vi "Delete Image.vi"(8 "Error In":errorcluster, 11 "Image Object":T1={"Device ID"=0, "Memeroy ID"=0, "Image Parameters"={"Channel Order"=enum."CL_LUMINANCE (Grayscale)", "Dimension"={"Depth"=1, "Height"=1, "Width"=1}, "Data Type"=enum."32f", "Offset"={"X"=0, "Y"=0, "Z"=0}}} {"Image Parameters"."Dimension"."Width" min=1; "Image Parameters"."Dimension"."Height" min=1; "Image Parameters"."Dimension"."Depth" min=1}) -> (0 "Error Out":errorcluster, 3 "Device Out":T2)   [LabVIEW 2012]
doc: "Deletes allocated memory on a device. It is best to call this at the end to avoid memory fragmentation due to constantly allocating and deleting memory."
uses:
  Non-User VIs/Controls/Device ID.ctl
  Non-User VIs/Controls/Image Object.ctl
  Non-User VIs/Controls/Memory ID.ctl
  Non-User VIs/Controls/Image Parameters.ctl
  Non-User VIs/Images/Channel Order.ctl
  User Controls/Array Dimensions.ctl
  Non-User VIs/Images/Data Type.ctl
  User Controls/Offset.ctl
  Non-User VIs/Error Checking/Add Error Functional Global.vi
  OpenCLV x64.lvlib
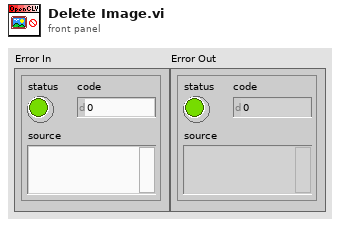
[diagram p1: front panel]
types:
  T1 = typedef "OpenCLV x64.lvlib/Image Object.ctl" = cluster{"Device ID":T2, "Memeroy ID":T3, "Image Parameters":T4}
  T2 = typedef "OpenCLV x64.lvlib/Device ID.ctl" = u64
  T3 = typedef "OpenCLV x64.lvlib/Memory ID.ctl" = u64
  T4 = typedef "OpenCLV x64.lvlib/Image Parameters.ctl" = cluster{"Channel Order":T5, "Dimension":T6, "Data Type":T7, "Offset":T8}
  T5 = typedef "OpenCLV x64.lvlib/Channel Order.ctl" = enum16{"CL_LUMINANCE (Grayscale)", "CL_INTENSITY (Opacity)", "CL_RGBA", "CL_ARGB", "CL_BGRA", "CL_RG", "CL_RA", "CL_R", "CL_A"}
  T6 = typedef "Array Dimensions.ctl" = cluster{"Depth":u64, "Height":u64, "Width":u64}
  T7 = typedef "OpenCLV x64.lvlib/Data Type.ctl" = enum16{"32f", "u8", "u16", "u32", "i8", "i16", "i32"}
  T8 = typedef "Offset.ctl" = cluster{"X":u64, "Y":u64, "Z":u64}
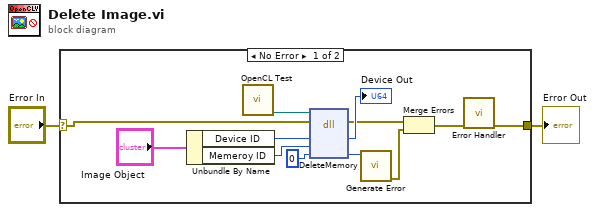
[diagram p0: block diagram]
diagram:
  n1 = case shown="No Error" "Error In" {
    selector: "Error In" -> [w3 w15]
    tunnel: [w8 w15] -> w1
    frame No Error {
      n2 = Unbundle By Name("Image Object") -> ("Device ID"=w11:T2, "Memeroy ID"=w12:T3)
      n3 = call "OpenCL Test.vi"() -> ("DLL To Use"=w9:path)  [unwired: 11 in]
      n4 = dll-call lib="C:/Users/bme-amcelroy-la/Desktop/OpenCLV/trunk/OpenCLV_x64_1.0/OpenCLV_x64.dll" fn="DeleteMemory"(path in=w9, error in=w3, "Device"=w11, "Device Memory"=w12, "Error"=0) -> (error out=w5:errorcluster, "Device"=→"Device Out":u64, "Error"=w13:i32)  [unwired: 3 in, 1 out]
      n5 = call "Generate Error.vi"("Error"=w13) -> ("error out"=w7:errorcluster)  [unwired: 10 in]
      n6 = Merge Errors(w5, w7) -> (w6:errorcluster)
      n7 = call-poly "Error Handler.vi"("Error In"=w6) -> ("Error Out"=w8:errorcluster)  [unwired: 10 in]
    }
    frame Error {
    }
  }
  "Error Out" <- w1
